vi "Write duration_sec.vi"(8 "error in (no error)":errorcluster, 10 "duration_sec":dbl, 11 "PCAP Frame Logger in":refnum<class "PCAP Frame Logger.lvclass">) -> (0 "error out":errorcluster, 3 "PCAP Frame Logger out":refnum<class "PCAP Frame Logger.lvclass">)   [LabVIEW 2020, in "AIM ARINC 664 Engine.lvlib" / "Implementation.lvlib" / "PCAP Frame Logger.lvclass"]
uses:
  PCAP Frame Logger.lvclass
  PCAP Frame Logger.lvclass/PCAP Frame Logger.ctl
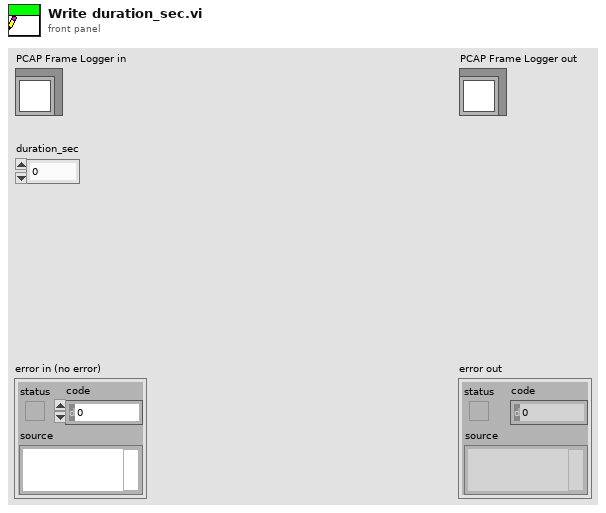
[diagram p1: front panel]
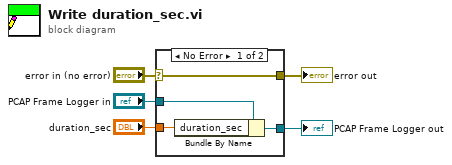
[diagram p0: block diagram]
diagram:
  n1 = case shown="No Error" "error in (no error)" {
    selector: "error in (no error)" -> [w9 w10]
    tunnel: [w9 w10] -> w4
    tunnel: [w7 w11] -> w2
    tunnel: "PCAP Frame Logger in" -> [w8 w11]
    tunnel: "duration_sec" -> [w6 _]
    frame No Error {
      n2 = Bundle By Name(cluster=w8, "duration_sec"=w6) -> (w7:refnum<class "PCAP Frame Logger.lvclass">)
    }
    frame Error {
    }
  }
  "error out" <- w4
  "PCAP Frame Logger out" <- w2
